vi "Save-Load Sys Config.vi"(7 "Standalone viewer?":bool, 8 "error in":errorcluster, 9 "System config to save":T1={"XY Stage"={"COM port"="", "XY stage available"=FALSE, "Baudrate"=0, "Type"=""}, "DAQ FPGA"={"Target"="RIO0", "input card type"=enum."AC Card", "Ref"=refnum, "Clock Freq (MHz) "=200.0, "Samples Wait after Trigger"=5080, "AOD fill"=4900, "StartupDelay"=0, "Slip Cycle (clock cycles)"=600000, "Add Cycle"=TRUE}, "Control system"={"Contrl Sys Available Ind"=FALSE, "Control system.FPGA Type"=enum."Virtex 7", "Control system.Network adapter name"="", "Control system.MAC address"="", "Control system.Ethernet Port"=3, "Ethernet opened"=FALSE, "Ctrl FPGA Clock (MHz)"=240.0, "AOD 1 Amplitude"=0, "AOD 2 Amplitude"=0, "AOD 3 Amplitude"=0, "AOD 4 Amplitude"=0, "AOD 5 Amplitude"=0, "AOD 6 Amplitude"=0, "Data Time Interval (ns)"=0.0, "T0 (ns)"=0.0, "Ta (ns)"=0.0}, "Encoder"={"IP address"="224.0.1.103", "Port"=7000, "Wheel radius (cm)"=16.0, "Encoder Trigger"=""}, "DAQmx Chan"={"Pockels AO"="", "Hard shutter AO"="", "PMT AOs"="", "Galvo AOs"="", "Power meter AI"=""}, "Computer MAC address"="", "Cam VidRec"={"DO flag-Video record"="", "DO flag-Trial start"=""}, "Externalise Triggers"=FALSE, "MC Supported"=FALSE, "Laser wavelength (nm)"=920.0} {"Laser wavelength (nm)" min=800.0 max=1080.0 step=1.0; "Encoder"."Wheel radius (cm)" format="%#_13g"; "Control system"."Control system.Ethernet Port" min=0 max=2048 step=1; "Control system"."Ctrl FPGA Clock (MHz)" min=80.0 max=500.0 step=1.0; "Control system"."Data Time Interval (ns)" min=0.0 max=2048.0 step=1.0; "Control system"."Ta (ns)" min=0.0 max=2048.0 step=1.0; "Control system"."T0 (ns)" min=0.0 max=2048.0 step=1.0; "Control system"."AOD 6 Amplitude" min=0 max=2048 step=1; "Control system"."AOD 5 Amplitude" min=0 max=2048 step=1; "Control system"."AOD 4 Amplitude" min=0 max=2048 step=1; "Control system"."AOD 3 Amplitude" min=0 max=2048 step=1; "Control system"."AOD 2 Amplitude" min=0 max=2048 step=1; "Control system"."AOD 1 Amplitude" min=0 max=2048 step=1}, 11 "Function":T11=enum."Load from file") -> (0 "error out":errorcluster, 1 "Loaded System config":T1={"XY Stage"={"COM port"="", "XY stage available"=FALSE, "Baudrate"=0, "Type"=""}, "DAQ FPGA"={"Target"="RIO0", "input card type"=enum."AC Card", "Ref"=refnum, "Clock Freq (MHz) "=200.0, "Samples Wait after Trigger"=5080, "AOD fill"=4900, "StartupDelay"=0, "Slip Cycle (clock cycles)"=600000, "Add Cycle"=TRUE}, "Control system"={"Contrl Sys Available Ind"=FALSE, "Control system.FPGA Type"=enum."Virtex 7", "Control system.Network adapter name"="", "Control system.MAC address"="", "Control system.Ethernet Port"=3, "Ethernet opened"=FALSE, "Ctrl FPGA Clock (MHz)"=240.0, "AOD 1 Amplitude"=0, "AOD 2 Amplitude"=0, "AOD 3 Amplitude"=0, "AOD 4 Amplitude"=0, "AOD 5 Amplitude"=0, "AOD 6 Amplitude"=0, "Data Time Interval (ns)"=0.0, "T0 (ns)"=0.0, "Ta (ns)"=0.0}, "Encoder"={"IP address"="224.0.1.103", "Port"=7000, "Wheel radius (cm)"=16.0, "Encoder Trigger"=""}, "DAQmx Chan"={"Pockels AO"="", "Hard shutter AO"="", "PMT AOs"="", "Galvo AOs"="", "Power meter AI"=""}, "Computer MAC address"="", "Cam VidRec"={"DO flag-Video record"="", "DO flag-Trial start"=""}, "Externalise Triggers"=FALSE, "MC Supported"=FALSE, "Laser wavelength (nm)"=920.0} {"Laser wavelength (nm)" min=800.0 max=1080.0 step=1.0; "Encoder"."Wheel radius (cm)" format="%#_13g"; "Control system"."Control system.Ethernet Port" min=0 max=2048 step=1; "Control system"."Ctrl FPGA Clock (MHz)" min=80.0 max=500.0 step=1.0; "Control system"."Data Time Interval (ns)" min=0.0 max=2048.0 step=1.0; "Control system"."Ta (ns)" min=0.0 max=2048.0 step=1.0; "Control system"."T0 (ns)" min=0.0 max=2048.0 step=1.0; "Control system"."AOD 6 Amplitude" min=0 max=2048 step=1; "Control system"."AOD 5 Amplitude" min=0 max=2048 step=1; "Control system"."AOD 4 Amplitude" min=0 max=2048 step=1; "Control system"."AOD 3 Amplitude" min=0 max=2048 step=1; "Control system"."AOD 2 Amplitude" min=0 max=2048 step=1; "Control system"."AOD 1 Amplitude" min=0 max=2048 step=1})   [LabVIEW 2020]
uses:
  <vilib>/Utility/config.llb/NI_LVConfig.lvlib
  Typedefs/Which path.ctl
  Typedefs/XY Stage config cluster.ctl
  <vilib>/userDefined/High Color/nirio_resource_hc.ctl
  RIG-SPECIFIC FILES/FPGA Refs/FPGA Ref.ctl
  Typedefs/DAQ FPGA config cluster.ctl
  Typedefs/DAQmx physical channels cluster.ctl
  Typedefs/CTRL system config cluster.ctl
  Typedefs/Sys Configuration.ctl
  Typedefs/Save-Load enum.ctl
  Typedefs/FPGA input type AC-DC.ctl
  Typedefs/Encoder config cluster.ctl
  Typedefs/Cam VidRec HW config setup cluster.ctl
panel:
  # "THIS VI HAS BEEN PHASED OUT"
  # "<--- The \"PMT AOs\" DAQmx string will always contain\n                       2 channels is this format: PXI1Slot4/ao2:3"
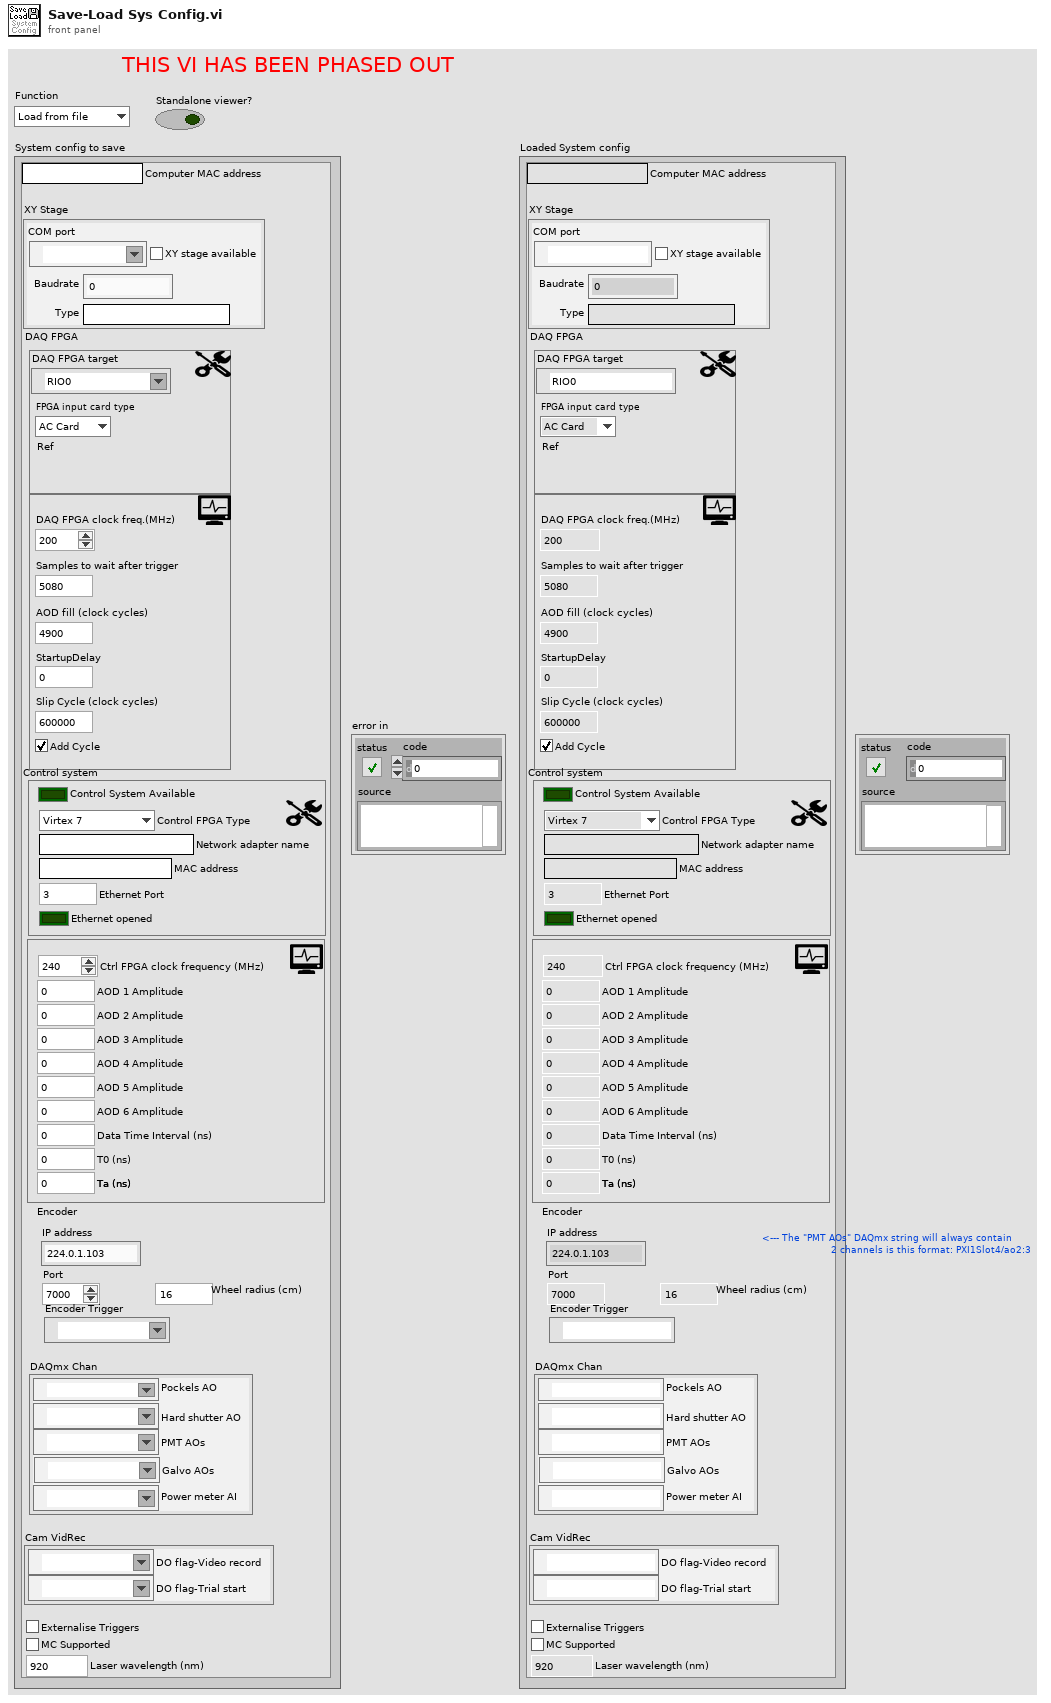
[diagram p1: front panel]
types:
  T1 = typedef "Sys Configuration.ctl" = cluster{"XY Stage":T2, "DAQ FPGA":T3, "Control system":T7, "Encoder":T8, "DAQmx Chan":T9, "Computer MAC address":string, "Cam VidRec":T10, "Externalise Triggers":bool, "MC Supported":bool, "Laser wavelength (nm)":dbl}
  T2 = typedef "XY Stage config cluster.ctl" = cluster{"COM port":refnum<visa-resource-name>, "XY stage available":bool, "Baudrate":i32, "Type":string}
  T3 = typedef "DAQ FPGA config cluster.ctl" = cluster{"Target":T4, "input card type":T5, "Ref":T6, "Clock Freq (MHz) ":dbl, "Samples Wait after Trigger":u16, "AOD fill":u16, "StartupDelay":i32, "Slip Cycle (clock cycles)":u32, "Add Cycle":bool}
  T4 = typedef "nirio_resource_hc.ctl" = tag
  T5 = typedef "FPGA input type AC-DC.ctl" = enum16{"AC Card", "DC Card"}
  T6 = typedef "FPGA Ref.ctl" = refnum<k20>
  T7 = typedef "CTRL system config cluster.ctl" = cluster{"Contrl Sys Available Ind":bool, "Control system.FPGA Type":enum16{"Virtex 5", "Virtex 7"}, "Control system.Network adapter name":string, "Control system.MAC address":string, "Control system.Ethernet Port":i16, "Ethernet opened":bool, "Ctrl FPGA Clock (MHz)":dbl, "AOD 1 Amplitude":i16, "AOD 2 Amplitude":i16, "AOD 3 Amplitude":i16, "AOD 4 Amplitude":i16, "AOD 5 Amplitude":i16, "AOD 6 Amplitude":i16, "Data Time Interval (ns)":dbl, "T0 (ns)":dbl, "Ta (ns)":dbl}
  T8 = typedef "Encoder config cluster.ctl" = cluster{"IP address":string, "Port":u16, "Wheel radius (cm)":dbl, "Encoder Trigger":tag}
  T9 = typedef "DAQmx physical channels cluster.ctl" = cluster{"Pockels AO":tag, "Hard shutter AO":tag, "PMT AOs":tag, "Galvo AOs":tag, "Power meter AI":tag}
  T10 = typedef "Cam VidRec HW config setup cluster.ctl" = cluster{"DO flag-Video record":tag, "DO flag-Trial start":tag}
  T11 = typedef "Save-Load enum.ctl" = enum16{"Save to file", "Load from file", "Compare from file", "Save Backup"}
  T12 = typedef "Which path.ctl" = enum16{"Configuration Files", "Calibration Files", "Images", "Setup.ini", "Loaded User profile.ini", "User's-Previous session.ini", "New user profile.ini", "Selected User profile.ini", "User profiles folder", "Power meter scaling.txt", "FOV Cal.ini", "Calibration.ini"}
  T13 = typedef "NI_LVConfig.lvlib/Config Data RefNum.ctl" = refnum<k1>
  T14 = typedef "Ini file interface (DBL).ctl" = cluster{"key":string, "Save?":bool, "Default":dbl}[]
  T15 = typedef "Ini file interface (String).ctl" = cluster{"key":string, "Save?":bool, "Default":string}[]
  T16 = typedef "Ini file interface (Boolean).ctl" = cluster{"key":string, "Save?":bool, "Default":bool}[]
  T17 = typedef "Sys Configuration.ctl" = cluster{"XY Stage":T18, "DAQ FPGA":T3, "Control system":T7, "Encoder":T8, "DAQmx Chan":T9, "Computer MAC address":string, "Cam VidRec":T10, "Externalise Triggers":bool, "MC Supported":bool, "Laser wavelength (nm)":dbl}
  T18 = typedef "XY Stage config cluster.ctl" = cluster{"COM port":refnum<visa-resource-name>, "Baudrate":i32, "Type":string}
  T19 = typedef "Hardware Configuration settings.ctl" = cluster{"Dev. PC":bool, "Swap XY on stage":bool, "No of AOD":u8, "MC Supported":bool, "Axial MC":bool, "Computer MAC address":string, "Externalise Triggers":bool, "Trigger HW config":T20, "DAQmx Chan":T9, "XY stage available":bool, "XY Stage":T2, "Z stage available":bool, "Z Stage config cluster":T21, "Encoder available":bool, "Encoder":T22, "VidRec available":bool, "Cam VidRec":T23, "Laser Power Control HW config":T24, "Laser 1 available":bool, "Laser 1 config cluster":T25, "Prechirper 1 available":bool, "Prechirper 1 config cluster":T26, "Control system.FPGA available?":bool, "Control Sys. HW config":T27, "DAQ FPGA HW Config":T28}
  T20 = typedef "Triggers HW config.ctl" = cluster{"Available Device List":i32, "Device Address":string}
  T21 = typedef "Z Stage config cluster.ctl" = cluster{"COM port":refnum<visa-resource-name>, "Z stage available":bool, "Baudrate":i32, "Type":string}
  T22 = typedef "Encoder config cluster.ctl" = cluster{"IP address":string, "Port":u16, "Encoder available":bool, "Wheel radius (cm)":dbl, "Encoder Trigger":tag}
  T23 = typedef "Cam VidRec HW config setup cluster.ctl" = cluster{"DO flag-Video record":tag, "DO flag-Trial start":tag, "VidRec available":bool}
  T24 = typedef "Laser Power Control HW config.ctl" = cluster{"Laser Power Control":string, "Laser Power Modulation Control":enum16{"NI", "FPGA"}}
  T25 = typedef "Laser 1 config cluster.ctl" = cluster{"COM port":refnum<visa-resource-name>, "Laser 1 available":bool, "Baud Rate":i32, "Type":string}
  T26 = typedef "PreChirper 1 config cluster.ctl" = cluster{"Type":string, "Baud Rate":i32, "Prechirper 1 available":bool, "COM port":refnum<visa-resource-name>}
  T27 = typedef "Control Sys HW config cluster.ctl" = cluster{"Control system.FPGA available?":bool, "Control system.FPGA Type":enum16{"Virtex 5", "Virtex 7"}, "Control system.Network adapter name":string, "Control system.MAC address":string, "Control system.Ethernet Port":u32, "Control system.Ethernet Port Opened":bool}
  T28 = typedef "DAQ FPGA HW config cluster.ctl" = cluster{"FGPA Ref":T6, "Target":T4, "input card type":T5}
  T29 = typedef "Hardware Configuration settings.ctl" = cluster{"Dev. PC":bool, "Swap XY on stage":bool, "No of AOD":u8, "MC Supported":bool, "Axial MC":bool, "Computer MAC address":string, "Externalise Triggers":bool, "Trigger HW config":T20, "DAQmx Chan":T9, "XY stage available":bool, "XY Stage":T18, "Z stage available":bool, "Z Stage config cluster":T30, "Encoder available":bool, "Encoder":T8, "VidRec available":bool, "Cam VidRec":T10, "Laser Power Control HW config":T24, "Laser 1 available":bool, "Laser 1 config cluster":T31, "Prechirper 1 available":bool, "Prechirper 1 config cluster":T32, "Control system.FPGA available?":bool, "Control Sys. HW config":T33, "DAQ FPGA HW Config":T28, "PMT Voltage Range":T34}
  T30 = typedef "Z Stage config cluster.ctl" = cluster{"COM port":refnum<visa-resource-name>, "Baudrate":i32, "Type":string}
  T31 = typedef "Laser 1 config cluster.ctl" = cluster{"COM port":refnum<visa-resource-name>, "Baud Rate":i32, "Type":string}
  T32 = typedef "PreChirper 1 config cluster.ctl" = cluster{"Type":string, "Baud Rate":i32, "COM port":refnum<visa-resource-name>}
  T33 = typedef "Control Sys HW config cluster.ctl" = cluster{"Control system.FPGA Type":enum16{"Virtex 5", "Virtex 7"}, "Control system.Network adapter name":string, "Control system.MAC address":string, "Control system.Ethernet Port":u32, "Control system.Ethernet Port Opened":bool}
  T34 = typedef "PMT Voltage Range.ctl" = cluster{"PMT Voltage Lower Limit":dbl, "PMT Voltage Upper Limit":dbl}
  T35 = cluster{"key":string, "Save?":bool, "Default":dbl}
  T36 = cluster{"key":string, "Save?":bool, "Default":dbl}[]
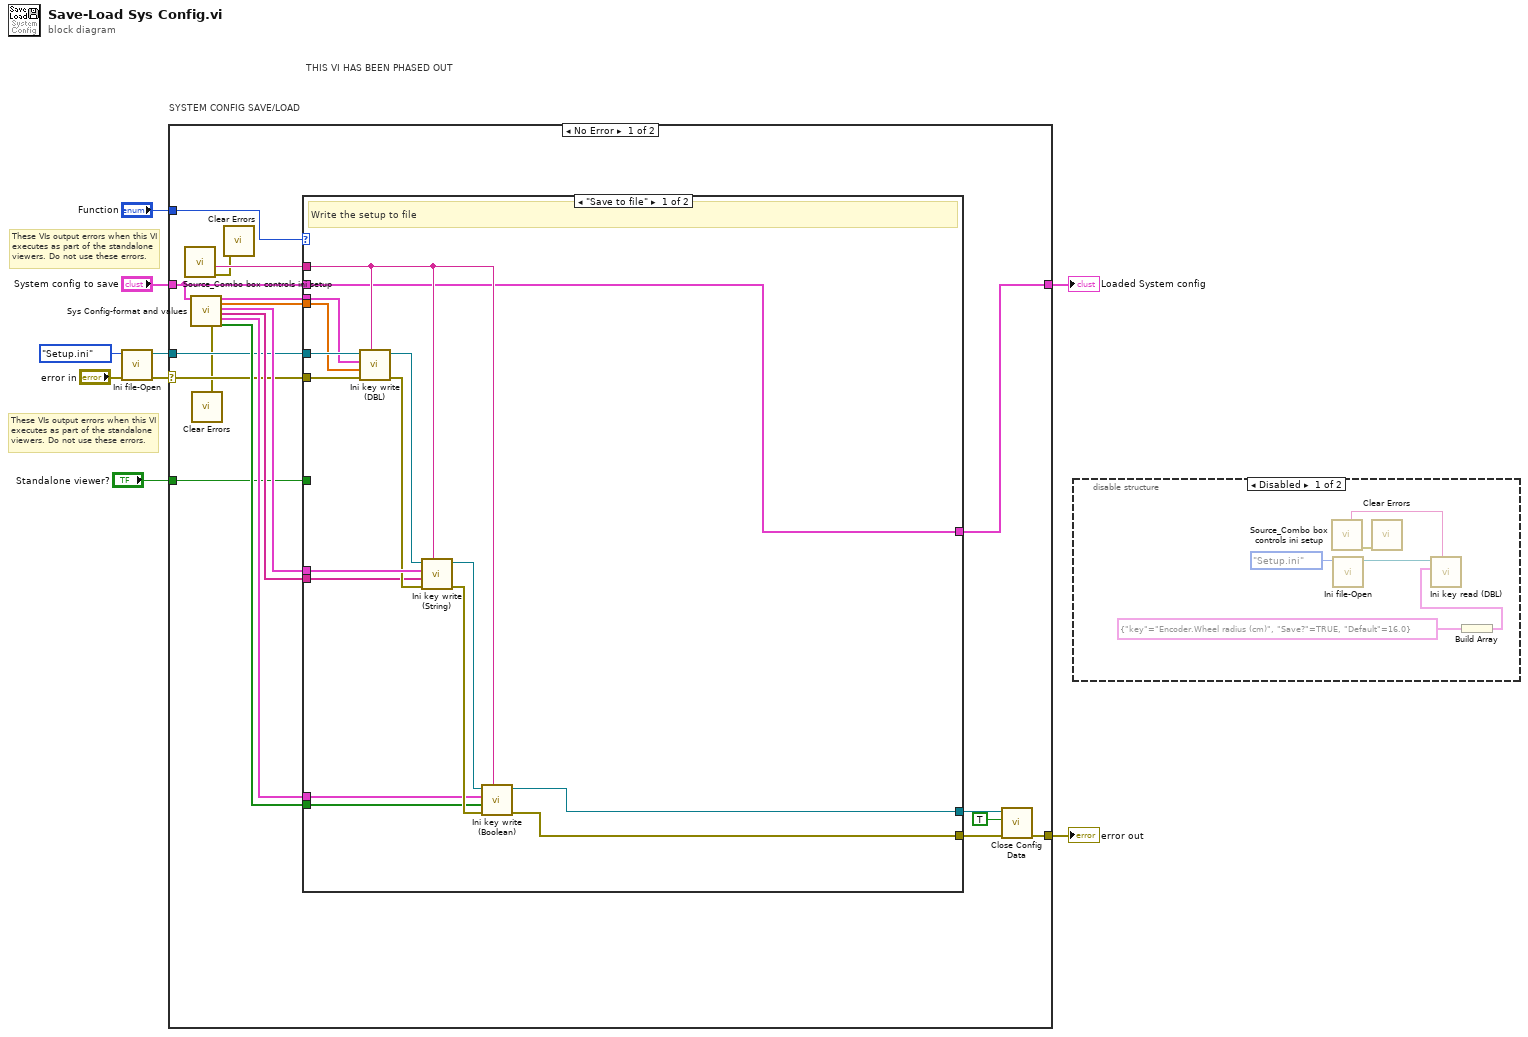
[diagram p0: block diagram]
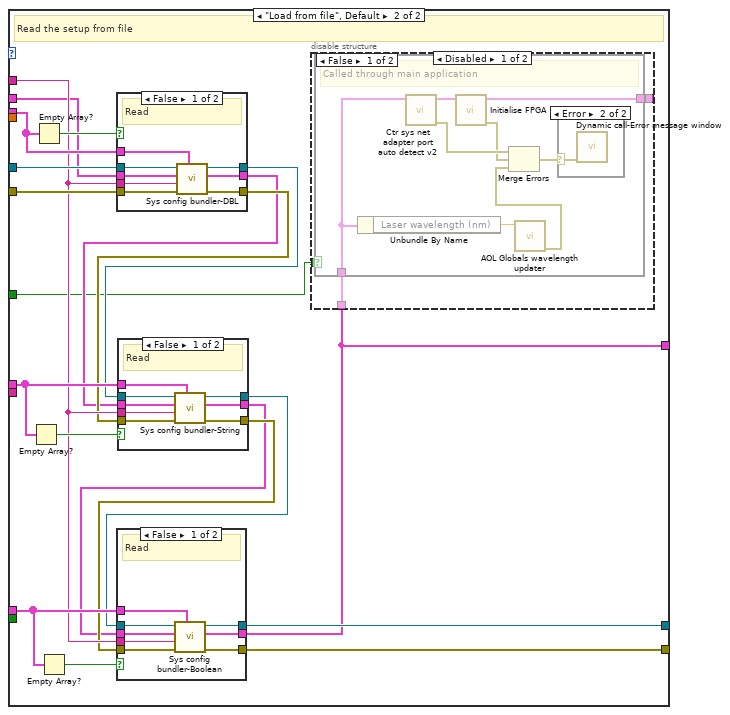
[diagram p3: hidden frame]
diagram:
  # "THIS VI HAS BEEN PHASED OUT"
  # "These VIs output errors when this VI executes as part of the standalone viewers. Do not use these errors."
  # "These VIs output errors when this VI executes as part of the standalone viewers. Do not use these errors."
  n1 = call "Ini file-Open.vi"("Error In"="error in", "Which file?"=Which_path."Setup.ini") -> ("error out"=w5:errorcluster, "User profile ini file ref"=w3:T13)  [unwired: 6 in, 2 out]
  n2 = case "SYSTEM CONFIG SAVE/LOAD" shown="No Error" w5 {
    selector: w5 -> [w18 w112]
    tunnel: [w16 w112] -> w2
    tunnel: "System config to save" -> [w26 w111]
    tunnel: [w10 w111] -> w8
    tunnel: "Function" -> [w19 _]
    tunnel: w3 -> [w17 _]
    tunnel: "Standalone viewer?" -> [w11 _]
    frame No Error {
      n3 = call "Source_Combo box controls ini setup.vi"() -> ("error out"=w13:errorcluster, "Section name"=w14:string)  [unwired: 9 in, 1 out]
      n4 = call "Sys Config-format and values.vi"("System Config"=w26) -> ("error out"=w12:errorcluster, "Keys setup.DBL"=w25:T14, "Values.DBL"=w24:dbl[], "Keys setup.String"=w23:T15, "Values.Strings"=w22:string[], "Keys setup.Boolean"=w21:T16, "Values.Boolean"=w20:bool[])  [unwired: 12 in]
      n5 = call <vilib>:"Clear Errors.vi"("error in (no error)"=w12) -> ()  [unwired: 5 in, 2 out]
      n6 = call <vilib>:"Clear Errors.vi"("error in (no error)"=w13) -> ()  [unwired: 5 in, 2 out]
      n7 = case shown="\"Save to file\"" w19 {
        tunnel: [w31 w59] -> w15
        tunnel: [w30 w60] -> w27
        tunnel: w18 -> [w43 w61]
        tunnel: w17 -> [w44 w64]
        tunnel: w14 -> [w33 w54]
        tunnel: w25 -> [w41 w63]
        tunnel: w24 -> [w42 _]
        tunnel: w20 -> [w32 _]
        tunnel: w21 -> [w34 w58]
        tunnel: w22 -> [w37 _]
        tunnel: w23 -> [w40 w55]
        tunnel: w26 -> [w29 w49]
        tunnel: w11 -> [_ w46]
        tunnel: [w29 w45] -> w10
        frame "Save to file" {
          # "Write the setup to file"
          n8 = call "Ini key write (DBL).vi"("Section"=w33, "error in (no error)"=w43, "Values (DBL)"=w42, "Ini file interface"=w41, "Ini file refnum in"=w44) -> ("error out"=w38:errorcluster, "Ini file refnum out"=w39:T13)  [unwired: 5 in]
          n9 = call "Ini key write (String).vi"("Section"=w33, "error in (no error)"=w38, "Values (String)"=w37, "Ini file interface"=w40, "Ini file refnum in"=w39) -> ("error out"=w35:errorcluster, "Ini file refnum out"=w36:T13)  [unwired: 5 in]
          n10 = call "Ini key write (Boolean).vi"("Section"=w33, "error in (no error)"=w35, "Values (Boolean)"=w32, "Ini file interface"=w34, "Ini file refnum in"=w36) -> ("error out"=w31:errorcluster, "Ini file refnum out"=w30:T13)  [unwired: 5 in]
        }
        frame "Load from file", Default {
          # "Read the setup from file"
          n11 = Empty Array?(array=w55) -> (empty?=w56:bool)
          n12 = Empty Array?(array=w63) -> (empty?=w62:bool)
          n13 = Empty Array?(array=w58) -> (empty?=w57:bool)
          n14 = case shown="False" w62 {
            tunnel: w64 -> [w107 w110]
            tunnel: [w106 w110] -> w50
            tunnel: [w105 w109] -> w51
            tunnel: w61 -> [w104 w109]
            tunnel: w54 -> [w102 _]
            tunnel: w63 -> [w103 _]
            tunnel: w49 -> [w101 w108]
            tunnel: [w100 w108] -> w48
            frame False {
              # "Read"
              n15 = call "Sys config bundler-DBL.vi"("Keys setup.DBL"=w103, "error in (no error)"=w104, "Section name"=w102, "System Config to save in"=w101, "Refnum in"=w107) -> ("error out"=w105:errorcluster, "System Config to save out"=w100:T17, "Refnum out"=w106:T13)  [unwired: 4 in]
            }
            frame True {
              # "No parametersof such type"
            }
          }
          n16 = case shown="False" w56 {
            tunnel: [w82 w88] -> w53
            tunnel: [w81 w87] -> w52
            tunnel: w55 -> [w84 _]
            tunnel: w50 -> [w85 w88]
            tunnel: w51 -> [w80 w87]
            tunnel: w54 -> [w83 _]
            tunnel: w48 -> [w79 w86]
            tunnel: [w78 w86] -> w47
            frame False {
              # "Read"
              n17 = call "Sys config bundler-String.vi"("Keys setup.String"=w84, "error in (no error)"=w80, "Section name"=w83, "System Config to save in"=w79, "Refnum in"=w85) -> ("error out"=w81:errorcluster, "System Config to save out"=w78:T1, "Refnum out"=w82:T13)  [unwired: 4 in]
            }
            frame True {
              # "No parametersof such type"
            }
          }
          n18 = case shown="False" w57 {
            tunnel: [w95 w99] -> w60
            tunnel: [w94 w98] -> w59
            tunnel: w58 -> [w91 _]
            tunnel: w53 -> [w96 w99]
            tunnel: w52 -> [w93 w98]
            tunnel: w54 -> [w92 _]
            tunnel: w47 -> [w90 w97]
            tunnel: [w89 w97] -> w45
            frame False {
              # "Read"
              n19 = call "Sys config bundler-Boolean.vi"("Keys setup.Boolean"=w91, "error in (no error)"=w93, "Section name"=w92, "System Config to save in"=w90, "Refnum in"=w96) -> ("error out"=w94:errorcluster, "System Config to save"=w89:T17, "Refnum out"=w95:T13)  [unwired: 4 in]
            }
            frame True {
              # "No parametersof such type"
            }
          }
          n20 = disable-structure shown="Disabled" {
            disable-tunnel: [w67 _] -> _
            disable-tunnel: w45 -> [w66 _]
            disable-tunnel: w46 -> [w65 _]
            frame Disabled {
              n21 = case shown="False" w65 {
                tunnel: [w71 w77] -> w67
                tunnel: w66 -> [w68 w77]
                frame False {
                  # "Called through main application"
                  n22 = Unbundle By Name(w68) -> ("Laser wavelength (nm)"=w69:dbl)
                  n23 = call "Ctr sys net adapter port auto detect v2.vi"("Hardware Configuration"=w68) -> ("error out"=w74:errorcluster, "Hardware Configuration O/P"=w75:T19)  [unwired: 8 in, 1 out]
                  n24 = call "Initialise FPGA.vi"("Hardware Resources in"=w75) -> ("error out"=w73:errorcluster, "Hardware Resources out"=w71:T29)  [unwired: 9 in]
                  n25 = call "AOL Globals wavelength updater.vi"("Laser wavelength (nm)"=w69) -> ("error out"=w70:errorcluster)  [unwired: 10 in]
                  n26 = Merge Errors(w74, w73, w70) -> (w72:errorcluster)
                  n27 = case shown="Error" w72 {
                    selector: w72 -> [_ w76]
                    frame No Error {
                    }
                    frame Error {
                      n28 = call "Dynamic call-Error message window.vi"("error in (no error)"=w76) -> ()  [unwired: 10 in, 1 out]
                    }
                  }
                }
                frame True {
                  # "Standalone viewer"
                }
              }
            }
            frame Enabled {
            }
          }
        }
      }
      n29 = call <vilib>:"Close Config Data.vi"("error in (no error)"=w15, "write file if changed (T)"=TRUE ("write configuration file? (F)"), "refnum"=w27) -> ("error out"=w16:errorcluster)  [unwired: 7 in, 1 out]
    }
    frame Error {
    }
  }
  "error out" <- w2
  "Loaded System config" <- w8
  n30 = disable-structure shown="Disabled" {
    frame Disabled {
      n31 = call "Source_Combo box controls ini setup.vi"() -> ("error out"=w113:errorcluster, "Section name"=w114:string)  [unwired: 9 in, 1 out]
      n32 = call "Ini file-Open.vi"("Which file?"=Which_path."Setup.ini") -> ("User profile ini file ref"=w117:T13)  [unwired: 7 in, 3 out]
      n33 = call <vilib>:"Clear Errors.vi"("error in (no error)"=w113) -> ()  [unwired: 5 in, 2 out]
      n34 = Build Array(T35 {"key"="Encoder.Wheel radius (cm)", "Save?"=TRUE, "Default"=16.0}) -> (w115:T36)
      n35 = call "Ini key read (DBL).vi"("Section name"=w114, "Parameter names & setup"=w115, "Ini file refnum in"=w117) -> ()  [unwired: 6 in, 3 out]
    }
    frame Enabled {
    }
  }
